vi "Resume.vi"(6 "nargs":i32, 10 "error in (no error)":errorcluster, 11 "Lua Thread in":refnum<class "Lua Thread.lvclass">) -> (1 "done?":bool, 2 "error out":errorcluster, 3 "Lua Thread out":refnum<class "Lua Thread.lvclass">, 4 "nresults":i32)   [LabVIEW 2020, in "Lua for LabVIEW.lvlib" / "Lua Thread.lvclass"]
doc: "Starts and resumes a coroutine in the given thread L.\n\nTo start a coroutine, you push onto the thread stack the main function plus any arguments; then you call lua_resume, with nargs being the number of arguments. This call returns when the coroutine suspends or finishes its execution. When it returns, the stack contains all values passed to lua_yield, or all values returned by the body function. lua_resume returns LUA_YIELD if the coroutine yields, LUA_OK if the coroutine finishes its execution without errors, or an error code in case of errors (see lua_pcall).\n\nIn case of errors, the stack is not unwound, so you can use the debug API over it. The error object is on the top of the stack.\n\nTo resume a coroutine, you remove any results from the last lua_yield, put on its stack only the values to be passed as results from yield, and then call lua_resume.\n\nThe parameter from represents the coroutine that is resuming L. If there is no such coroutine, this parameter can be NULL."
uses:
  Lua Thread.lvclass
  Lua Thread.lvclass/Lua Thread.ctl
  Lua/Lua.lvclass
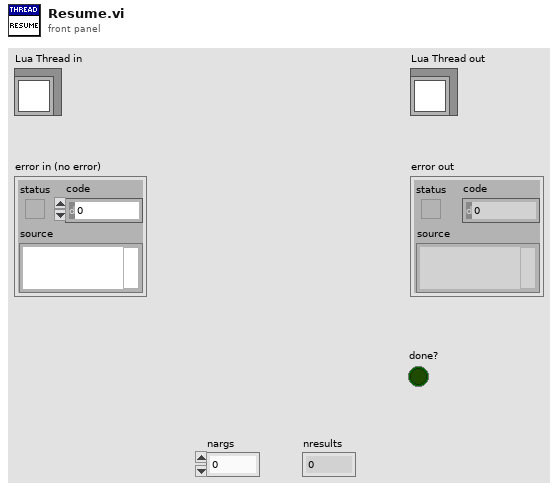
[diagram p1: front panel]
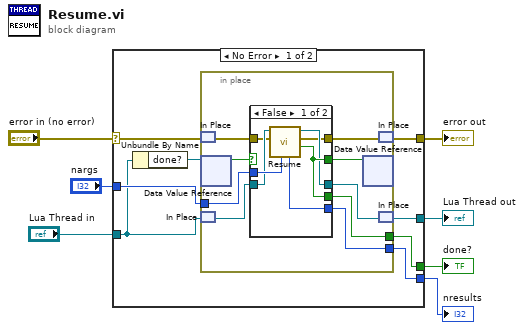
[diagram p0: block diagram]
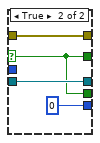
[diagram p2: hidden frame]
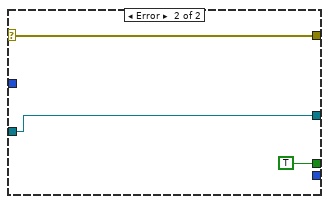
[diagram p3: hidden frame]
diagram:
  n1 = case shown="No Error" "error in (no error)" {
    selector: "error in (no error)" -> [w10 w38]
    tunnel: [w9 w38] -> w7
    tunnel: [w15 TRUE ("done?")] -> w6
    tunnel: [w14 _] -> w5
    tunnel: "nargs" -> [w13 _]
    tunnel: "Lua Thread in" -> [w11 w36]
    tunnel: [w8 w36] -> w1
    frame No Error {
      n2 = Unbundle By Name(w11) -> ("done?"=w12:refnum<data-value>)
      n3 = in-place {
        in-place-border: [w24] -> w15
        in-place-border: [w23] -> w14
        in-place-border: w13 -> [w22]
        n4 = in-place-match #1(w10) -> (w18:errorcluster)
        n5 = in-place-dvr #2(w12) -> (w21:bool)  [unwired: 1 out]
        n6 = in-place-match #3(w11) -> (w19:refnum<class "Lua Thread.lvclass">)
        n7 = case shown="False" w21 {
          selector: w21 -> [_ w34]
          tunnel: [w26 w33] -> w17
          tunnel: [w29 w34] -> w24
          tunnel: [w31 0 ("nresults")] -> w23
          tunnel: w22 -> [w30 _]
          tunnel: w19 -> [w28 w35]
          tunnel: [w29 w34] -> w20
          tunnel: [w27 w35] -> w16
          tunnel: w18 -> [w25 w33]
          frame False {
            n8 = call-parent "Resume.vi"("nargs"=w30, "error in (no error)"=w25, "Lua in"=w28) -> ("done?"=w29:bool, "error out"=w26:errorcluster, "Lua out"=w27:refnum<class "Lua Thread.lvclass">, "nresults"=w31:i32)  [unwired: 5 in]
          }
          frame True {
          }
        }
        n9 = in-place-dvr #2(w20) -> ()  [unwired: 2 out]
        n10 = in-place-match #1(w17) -> (w9:errorcluster)
        n11 = in-place-match #3(w16) -> (w8:refnum<class "Lua Thread.lvclass">)
      }
    }
    frame Error {
    }
  }
  "error out" <- w7
  "Lua Thread out" <- w1
  "nresults" <- w5
  "done?" <- w6
